vi "Controller to Joystick.vi"(10 "Controller Buttons":T1, 11 "Controller Axis":T11) -> (2 "Joystick Buttons":T1, 3 "Joystick Axis":T11)   [LabVIEW 2018]
uses:
  <vilib>/MakerHub/Xbox-One-Controller/Private/Type Defs/Indicators/All Axis Data.ctl
  <vilib>/MakerHub/Xbox-One-Controller/Private/Type Defs/Indicators/DPad Enum.ctl
  <vilib>/MakerHub/Xbox-One-Controller/Private/Type Defs/Indicators/All Buttons Visual.ctl
  <vilib>/MakerHub/Xbox-One-Controller/Private/Type Defs/Indicators/A.ctl
  <vilib>/MakerHub/Xbox-One-Controller/Private/Type Defs/Indicators/B.ctl
  <vilib>/MakerHub/Xbox-One-Controller/Private/Type Defs/Indicators/X.ctl
  <vilib>/MakerHub/Xbox-One-Controller/Private/Type Defs/Indicators/Y.ctl
  <vilib>/MakerHub/Xbox-One-Controller/Private/Type Defs/Indicators/Left Bumper.ctl
  <vilib>/MakerHub/Xbox-One-Controller/Private/Type Defs/Indicators/Right Bumper.ctl
  <vilib>/MakerHub/Xbox-One-Controller/Private/Type Defs/Indicators/View.ctl
  <vilib>/MakerHub/Xbox-One-Controller/Private/Type Defs/Indicators/Menu.ctl
  <vilib>/MakerHub/Xbox-One-Controller/Private/Type Defs/Indicators/Thumbstick.ctl
  <vilib>/MakerHub/Xbox-One-Controller/LMH-Xbox-One-Controller.lvlib
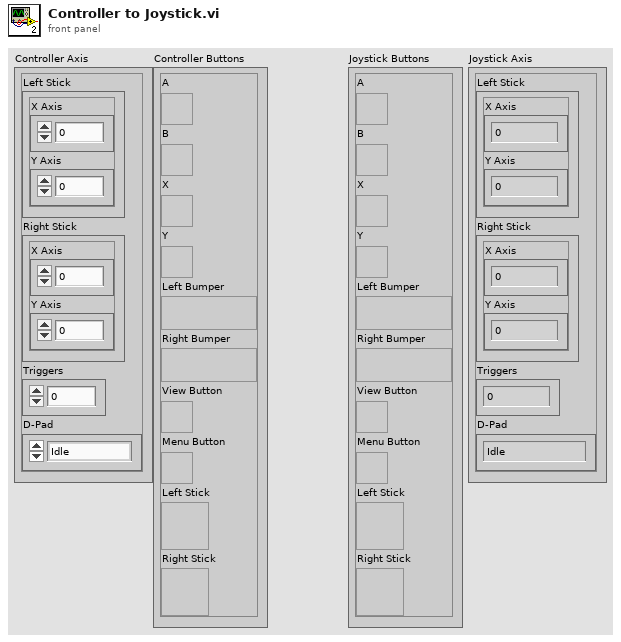
[diagram p1: front panel]
types:
  T1 = typedef "LMH-Xbox-One-Controller.lvlib/All Buttons Visual.ctl" = cluster{"A":T2, "B":T3, "X":T4, "Y":T5, "Left Bumper":T6, "Right Bumper":T7, "View Button":T8, "Menu Button":T9, "Left Stick":T10, "Right Stick":T10}
  T2 = typedef "LMH-Xbox-One-Controller.lvlib/A.ctl" = bool
  T3 = typedef "LMH-Xbox-One-Controller.lvlib/B.ctl" = bool
  T4 = typedef "LMH-Xbox-One-Controller.lvlib/X.ctl" = bool
  T5 = typedef "LMH-Xbox-One-Controller.lvlib/Y.ctl" = bool
  T6 = typedef "LMH-Xbox-One-Controller.lvlib/Left Bumper.ctl" = bool
  T7 = typedef "LMH-Xbox-One-Controller.lvlib/Right Bumper.ctl" = bool
  T8 = typedef "LMH-Xbox-One-Controller.lvlib/View.ctl" = bool
  T9 = typedef "LMH-Xbox-One-Controller.lvlib/Menu.ctl" = bool
  T10 = typedef "LMH-Xbox-One-Controller.lvlib/Thumbstick.ctl" = bool
  T11 = typedef "LMH-Xbox-One-Controller.lvlib/All Axis Data.ctl" = cluster{"Left Stick":cluster{"X Axis":i32, "Y Axis":i32}, "Right Stick":cluster{"X Axis":i32, "Y Axis":i32}, "Triggers":i32, "D-Pad":T12}
  T12 = typedef "LMH-Xbox-One-Controller.lvlib/DPad Enum.ctl" = enum16{"Idle", "Up", "Up / Right", "Right", "Down / Right", "Down", "Down / Left", "Left", "Up / Left"}
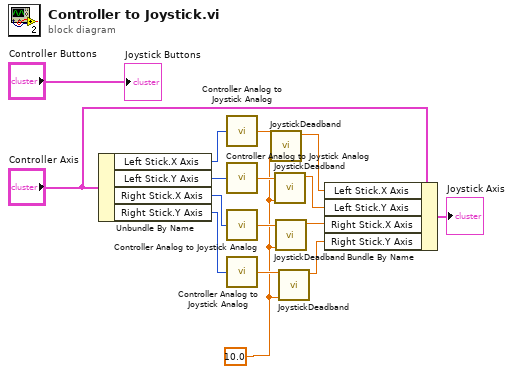
[diagram p0: block diagram]
diagram:
  w1 = 10.0
  n1 = Unbundle By Name("Controller Axis") -> ("Left Stick.X Axis"=w16:i32, "Left Stick.Y Axis"=w15:i32, "Right Stick.X Axis"=w14:i32, "Right Stick.Y Axis"=w13:i32)
  n2 = call "Controller Analog to Joystick Analog.vi"("Controller Value"=w16) -> ("Joystick Value"=w3:dbl)
  n3 = call "Controller Analog to Joystick Analog.vi"("Controller Value"=w15) -> ("Joystick Value"=w4:dbl)
  n4 = call "Controller Analog to Joystick Analog.vi"("Controller Value"=w14) -> ("Joystick Value"=w7:dbl)
  n5 = call "Controller Analog to Joystick Analog.vi"("Controller Value"=w13) -> ("Joystick Value"=w9:dbl)
  n6 = call "JoystickDeadband.vi"("Deadband %"=w1, "Joystick Value"=w3) -> ("Joystick Value"=w2:dbl)  [unwired: 9 in]
  n7 = call "JoystickDeadband.vi"("Deadband %"=w1, "Joystick Value"=w4) -> ("Joystick Value"=w5:dbl)  [unwired: 9 in]
  n8 = call "JoystickDeadband.vi"("Deadband %"=w1, "Joystick Value"=w7) -> ("Joystick Value"=w6:dbl)  [unwired: 9 in]
  n9 = call "JoystickDeadband.vi"("Deadband %"=w1, "Joystick Value"=w9) -> ("Joystick Value"=w8:dbl)  [unwired: 9 in]
  n10 = Bundle By Name(cluster="Controller Axis", "Left Stick.X Axis"=w2, "Left Stick.Y Axis"=w5, "Right Stick.X Axis"=w6, "Right Stick.Y Axis"=w8) -> (→"Joystick Axis":T11)
  "Joystick Buttons" <- "Controller Buttons"
